vi "Brain.vi"(8 "Index":T1={"N1"=18, "N2"=19, "N3"=4, "N4"=5, "V1"=8, "V2"=10, "V3"=10, "V4"=13, "CURRENT"=12, "Vsg"=1}, 9 "voltage":bool=TRUE, 10 "Conductance":T2(graph), 11 "Folder Path":path) -> (2 "Conductance 2":T2(graph))   [LabVIEW 2016]
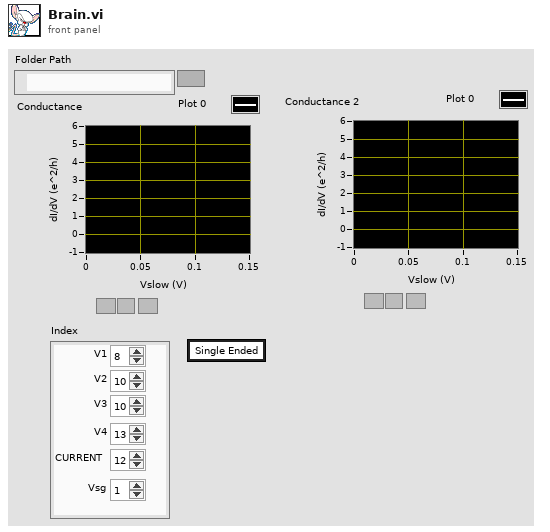
[diagram p1: front panel]
types:
  T1 = cluster{"N1":i32, "N2":i32, "N3":i32, "N4":i32, "V1":i32, "V2":i32, "V3":i32, "V4":i32, "CURRENT":i32, "Vsg":i32}
  T2 = cluster{"Vfast":dbl[], "Decimated Array":dbl[]}[]
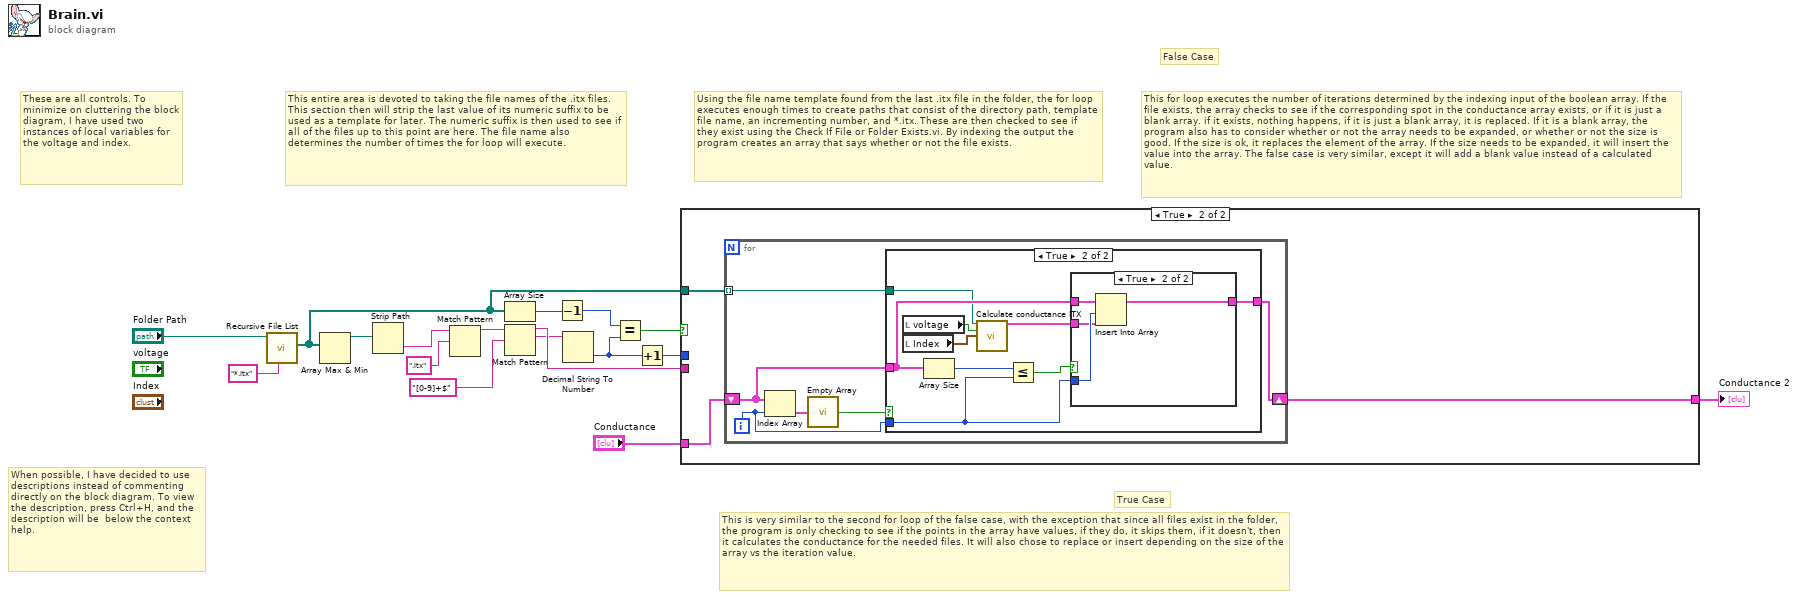
[diagram p0: block diagram]
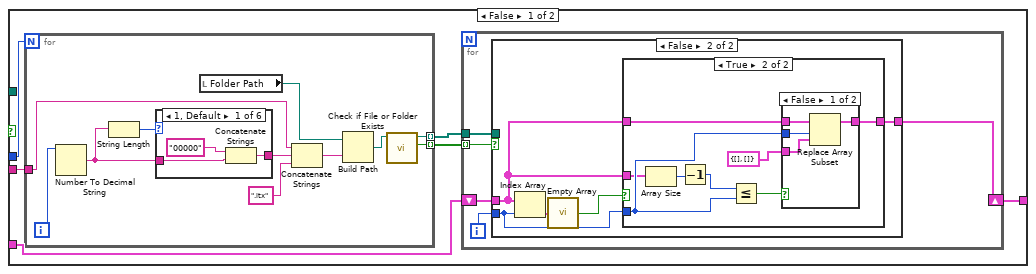
[diagram p2: hidden frame]
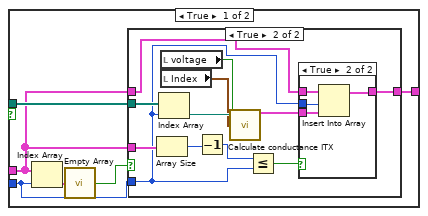
[diagram p3: hidden frame]
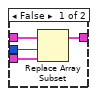
[diagram p5: hidden frame]
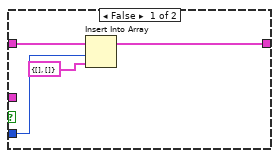
[diagram p6: hidden frame]
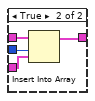
[diagram p7: hidden frame]
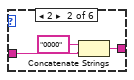
[diagram p8: hidden frame]
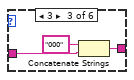
[diagram p9: hidden frame]
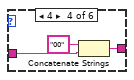
[diagram p10: hidden frame]
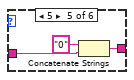
[diagram p11: hidden frame]
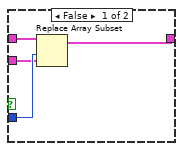
[diagram p14: hidden frame]
diagram:
  # "This is very similar to the second for loop of the false case, with the exception that since all files exist in the folder, the program is only checking to see if the points in the array have values, if they do, it skips them, if it doesn't, then it calculates the conductance for the needed files. It will also chose to replace or insert depending on the size of the array vs the iteration value."
  # "True Case"
  # "This for loop executes the number of iterations determined by the indexing input of the boolean array. If the file exists, the array checks to see if the corresponding spot in the conductance array exists, or if it is just a blank array. if it exists, nothing happens, if it is just a blank array, it is replaced. If it is a blank array, the program also has to consider whether or not the array needs to be expanded, or whether or not the size is good. If the size is ok, it replaces the element of the array. If the size needs to be expanded, it will insert the value into the array. The false case is very similar, except it will add a blank value instead of a calculated value."
  # "Using the file name template found from the last .itx file in the folder, the for loop executes enough times to create paths that consist of the directory path, template file name, an incrementing number, and *.itx. These are then checked to see if they exist using the Check If File or Folder Exists.vi. By indexing the output the program creates an array that says whether or not the file exists."
  # "False Case"
  # "This entire area is devoted to taking the file names of the .itx files. This section then will strip the last value of its numeric suffix to be used as a template for later. The numeric suffix is then used to see if all of the files up to this point are here. The file name also determines the number of times the for loop will execute."
  # "When possible, I have decided to use descriptions instead of commenting directly on the block diagram. To view the description, press Ctrl+H, and the description will be  below the context help."
  # "These are all controls. To minimize on cluttering the block diagram, I have used two instances of local variables for the voltage and index."
  n1 = call <vilib>:"Recursive File List.vi"("pattern"="*.itx", "Folder Path"="Folder Path") -> ("All Files in Dir"=w2:path[])  [unwired: 6 in, 3 out]
  n2 = Array Max & Min(array=w2) -> (max value=w16:path)  [unwired: 3 out]
  n3 = Strip Path(path=w16) -> (name=w15:string)  [unwired: 1 out]
  n4 = Match Pattern(string=w15, regular expression=".itx") -> (before substring=w13:string)  [unwired: 1 in, 3 out]
  n5 = Array Size(array=w2) -> (size(s)=w10:i32)
  n6 = Match Pattern(string=w13, regular expression="[0-9]+$") -> (before substring=w5:string, match substring=w4:string)  [unwired: 1 in, 2 out]
  n7 = Decrement(x=w10) -> (x-1=w9:i32)
  n8 = Decimal String To Number(string=w4) -> (number=w7:i32)  [unwired: 2 in, 1 out]
  n9 = Equal?(x=w9, y=w7) -> (x = y?=w8:bool)
  n10 = Increment(x=w7) -> (x+1=w6:i32)
  n11 = case shown="True" w8 {
    tunnel: w6 -> [w23 _]
    tunnel: w5 -> [w22 _]
    tunnel: "Conductance" -> [w19 w110]
    tunnel: [w18 w108] -> w1
    tunnel: w2 -> [_ w109]
    frame False {
      n12 = for {
        N: w23 -> [_]
        tunnel: w22 -> [w88]
        tunnel: [w82] -> w21 mode=indexing
        tunnel: [w81] -> w20 mode=indexing
        i -> [w91]
        n13 = Number To Decimal String(number=w91) -> (decimal integer string=w89:string)  [unwired: 1 in]
        n14 = String Length(string=w89) -> (length=w90:i32)
        n15 = case shown="1, Default" w90 {
          tunnel: w89 -> [w94 w97 w100 w103 w106 w107]
          tunnel: [w92 w96 w99 w102 w105 w107] -> w87
          frame 1, Default {
            n16 = Concatenate Strings("00000" ("string"), w94) -> (w92:string)
          }
          frame 2 {
            n17 = Concatenate Strings("0000" ("string"), w97) -> (w96:string)
          }
          frame 3 {
            n18 = Concatenate Strings("000" ("string"), w100) -> (w99:string)
          }
          frame 4 {
            n19 = Concatenate Strings("00" ("string"), w103) -> (w102:string)
          }
          frame 5 {
            n20 = Concatenate Strings("0" ("string"), w106) -> (w105:string)
          }
          frame 6 {
          }
        }
        n21 = local read "Folder Path"() -> (w84:path)
        n22 = Concatenate Strings(w88, w87, ".itx" ("string")) -> (w85:string)
        n23 = Build Path(base path=w84, name or relative path=w85) -> (appended path=w83:path)
        n24 = call <vilib>:"Check if File or Folder Exists.vi"("path"=w83) -> ("file or folder exists?"=w82:bool, "dup path"=w81:path)  [unwired: 8 in, 1 out]
      }
      n25 = for {
        tunnel: w21 -> [w28] mode=indexing
        tunnel: w20 -> [w25]
        shift-right: [w24] -> w18
        shift-left: w19 -> [w27]
        i -> [w26]
        n26 = case shown="False" w28 {
          tunnel: w27 -> [w30 w56]
          tunnel: w26 -> [w32 w58]
          tunnel: w25 -> [w31 _]
          tunnel: [w29 w57] -> w24
          frame True {
            n27 = Index Array(array=w30, index=w32) -> (element=w34:cluster{"Vfast":dbl[], "Decimated Array":dbl[]})
            n28 = call "Empty Array.vi"("Cluster"=w34) -> ("Boolean"=w33:bool)  [unwired: 8 in]
            n29 = case shown="True" w33 {
              tunnel: w30 -> [_ w44]
              tunnel: w32 -> [_ w37]
              tunnel: w31 -> [_ w45]
              tunnel: w30 -> [w35 w36]
              tunnel: [w35 w40] -> w29
              frame False {
              }
              frame True {
                n30 = Array Size(array=w44) -> (size(s)=w47:i32)
                n31 = Index Array(array=w45, index=w37) -> (element=w43:path)
                n32 = local read "voltage"() -> (w39:bool)
                n33 = local read "Index"() -> (w38:T1)
                n34 = Decrement(x=w47) -> (x-1=w46:i32)
                n35 = call "Calculate conductance ITX.vi"("File or Folder Path"=w43, "single ended?"=w39, "index"=w38) -> ("A vs D"=w41:cluster{dbl[], dbl[]}[])  [unwired: 9 in, 3 out]
                n36 = Less Or Equal?(x=w46, y=w37) -> (x <= y?=w42:bool)
                n37 = case shown="True" w42 {
                  tunnel: w41 -> [w51 w54]
                  tunnel: w36 -> [w50 w55]
                  tunnel: w37 -> [w49 w53]
                  tunnel: [w48 w52] -> w40
                  frame False {
                    n38 = Replace Array Subset(array=w50, new element=w51, index=w49) -> (w48:T2)
                  }
                  frame True {
                    n39 = Insert Into Array(array=w55, index=w53, new element=w54) -> (w52:T2)
                  }
                }
              }
            }
          }
          frame False {
            n40 = Index Array(array=w56, index=w58) -> (element=w60:cluster{"Vfast":dbl[], "Decimated Array":dbl[]})
            n41 = call "Empty Array.vi"("Cluster"=w60) -> ("Boolean"=w59:bool)  [unwired: 8 in]
            n42 = case shown="True" w59 {
              tunnel: w58 -> [w62 w68]
              tunnel: w56 -> [w64 w69]
              tunnel: [w63 w67] -> w57
              tunnel: w56 -> [_ w66]
              frame False {
                n43 = Insert Into Array(array=w64, index=w62, new element=cluster{"Vfast":dbl[], "Decimated Array":dbl[]} {"Vfast"=[], "Decimated Array"=[]} ("x")) -> (w63:T2)
              }
              frame True {
                n44 = Array Size(array=w66) -> (size(s)=w72:i32)
                n45 = Decrement(x=w72) -> (x-1=w71:i32)
                n46 = Less Or Equal?(x=w71, y=w68) -> (x <= y?=w70:bool)
                n47 = case shown="False" w70 {
                  tunnel: w69 -> [w76 w80]
                  tunnel: w68 -> [w75 w79]
                  tunnel: [w74 w78] -> w67
                  tunnel: cluster{"Vfast":dbl[], "Decimated Array":dbl[]} {"Vfast"=[], "Decimated Array"=[]} ("x") -> [w73 w77]
                  frame False {
                    n48 = Replace Array Subset(array=w76, new element=w73, index=w75) -> (w74:T2)
                  }
                  frame True {
                    n49 = Insert Into Array(array=w80, index=w79, new element=w77) -> (w78:T2)
                  }
                }
              }
            }
          }
        }
      }
    }
    frame True {
      n50 = for {
        shift-right: [w111] -> w108
        shift-left: w110 -> [w112]
        tunnel: w109 -> [w114] mode=indexing
        i -> [w113]
        n51 = Index Array(array=w112, index=w113) -> (element=w116:cluster{"Vfast":dbl[], "Decimated Array":dbl[]})
        n52 = call "Empty Array.vi"("Cluster"=w116) -> ("Boolean"=w115:bool)  [unwired: 8 in]
        n53 = case shown="True" w115 {
          tunnel: w114 -> [_ w118]
          tunnel: w113 -> [_ w124]
          tunnel: w112 -> [w117 w121]
          tunnel: [w117 w122] -> w111
          frame False {
          }
          frame True {
            n54 = local read "voltage"() -> (w120:bool)
            n55 = local read "Index"() -> (w119:T1)
            n56 = Array Size(array=w121) -> (size(s)=w126:i32)
            n57 = call "Calculate conductance ITX.vi"("File or Folder Path"=w118, "single ended?"=w120, "index"=w119) -> ("A vs D"=w123:cluster{dbl[], dbl[]}[])  [unwired: 9 in, 3 out]
            n58 = Less Or Equal?(x=w126, y=w124) -> (x <= y?=w125:bool)
            n59 = case shown="True" w125 {
              tunnel: w121 -> [w130 w134]
              tunnel: w124 -> [w129 w133]
              tunnel: w123 -> [w128 w132]
              tunnel: [w127 w131] -> w122
              frame False {
                n60 = Replace Array Subset(array=w130, new element=w128, index=w129) -> (w127:T2)
              }
              frame True {
                n61 = Insert Into Array(array=w134, index=w133, new element=w132) -> (w131:T2)
              }
            }
          }
        }
      }
    }
  }
  "Conductance 2" <- w1
